vi "DUAL SINGLE GAUGE-Conver4Int.vi"(0 "String in":string) -> (6 "Wert 1 out":dbl format="%.4f", 8 "Wert 2 out":dbl format="%.4f", 10 "Wert 3 out":dbl format="%.4f", 15 "Wert4 out":dbl format="%.4f")   [LabVIEW 2010, in "Dual Gauge.lvlib"]
uses:
  Dual Gauge.lvlib
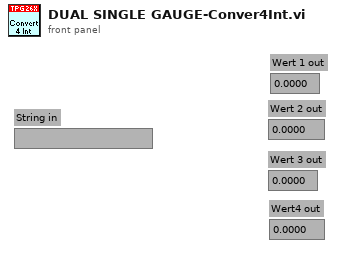
[diagram p1: front panel]
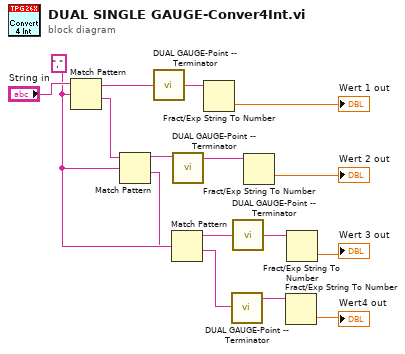
[diagram p0: block diagram]
diagram:
  w12 = "," ("regular expression")
  n1 = Match Pattern(string="String in", regular expression=w12) -> (before substring=w4:string, after substring=w8:string)  [unwired: 1 in, 2 out]
  n2 = Match Pattern(string=w8, regular expression=w12) -> (before substring=w13:string, after substring=w11:string)  [unwired: 1 in, 2 out]
  n3 = call "DUAL GAUGE-Point -- Terminator.vi"("Eingangstring"=w4) -> ("Ausgangstring"=w3:string)
  n4 = Match Pattern(string=w11, regular expression=w12) -> (before substring=w1:string, after substring=w6:string)  [unwired: 1 in, 2 out]
  n5 = call "DUAL GAUGE-Point -- Terminator.vi"("Eingangstring"=w13) -> ("Ausgangstring"=w10:string)
  n6 = Fract/Exp String To Number(string=w3) -> (number=→"Wert 1 out":dbl)  [unwired: 3 in, 1 out]
  n7 = call "DUAL GAUGE-Point -- Terminator.vi"("Eingangstring"=w6) -> ("Ausgangstring"=w9:string)
  n8 = call "DUAL GAUGE-Point -- Terminator.vi"("Eingangstring"=w1) -> ("Ausgangstring"=w2:string)
  n9 = Fract/Exp String To Number(string=w10) -> (number=→"Wert 2 out":dbl)  [unwired: 3 in, 1 out]
  n10 = Fract/Exp String To Number(string=w9) -> (number=→"Wert4 out":dbl)  [unwired: 3 in, 1 out]
  n11 = Fract/Exp String To Number(string=w2) -> (number=→"Wert 3 out":dbl)  [unwired: 3 in, 1 out]
